vi "XY Dialog - Update FP Settings With Persistent Data.vi"(7 "GraphData.System.Root":refnum<k24>, 8 "error in (no error)":errorcluster, 10 "References":T9, 11 "Persistent Data":T1={"Label"="", "Graph Props"={"Plots"=[], "Legend:Number of Rows"=0, "Scale Properties"={"X.Auto"=FALSE, "X.Min"=0.0, "X.Max"=0.0, "X.IgnoreTS"=FALSE, "X.Precision"=0, "X.Label:"="", "X.LabelVis"=FALSE, "X.DefLabel"=FALSE, "Y.Auto"=FALSE, "Y.Min"=0.0, "Y.Max"=0.0, "Y.Format"=0, "Y.Precision:"=0, "Y.Label:"="", "Y.LabelVis"=FALSE, "Y.DefLabel"=FALSE, "X.Format"=0}, "Legend:Visible"=TRUE, "BgColor"=0, "Last Plot Width"=0, "Resize"=FALSE}, "UDP Data"={"Decimation"=0, "UDP Buffer Size"=0, "History Length"=0.0, "Update Rate"=enum."15 Hz", "Channel Paths"=[], "Channel Names"=[]}} {"Graph Props"."Scale Properties"."X.Format" items=["Decimal", "Scientific", "Engineering", "Binary", "Octal", "Hexadecimal", "Relative Time", "Time and Date", "SI", "Automatic"]; "Graph Props"."Scale Properties"."Y.Precision:" items=["0", "1", "2", "3", "4", "5", "6", "7"]; "Graph Props"."Scale Properties"."Y.Format" items=["Decimal", "Scientific", "Engineering", "Binary", "Octal", "Hexadecimal", "Relative Time", "Time and Date", "SI", "Automatic"]; "Graph Props"."Scale Properties"."X.Precision" items=["0", "1", "2", "3", "4", "5", "6", "7"]}) -> (0 "error out":errorcluster)   [LabVIEW 2020, in "Workspace MultiY Graph.lvlib"]
uses:
  Workspace MultiY Graph.lvlib
  XY Dialog References.ctl
  XY Scale Precision.ctl
  XY Scale Format.ctl
  XY Persistent Data.ctl
  XY Graph Properties.ctl
  XY Plot Properties.ctl
  XY Scale Properties.ctl
  UDP Data.ctl
  Update Rate.ctl
  NationalInstruments.VeriStand.SystemStorage
  NationalInstruments.VeriStand
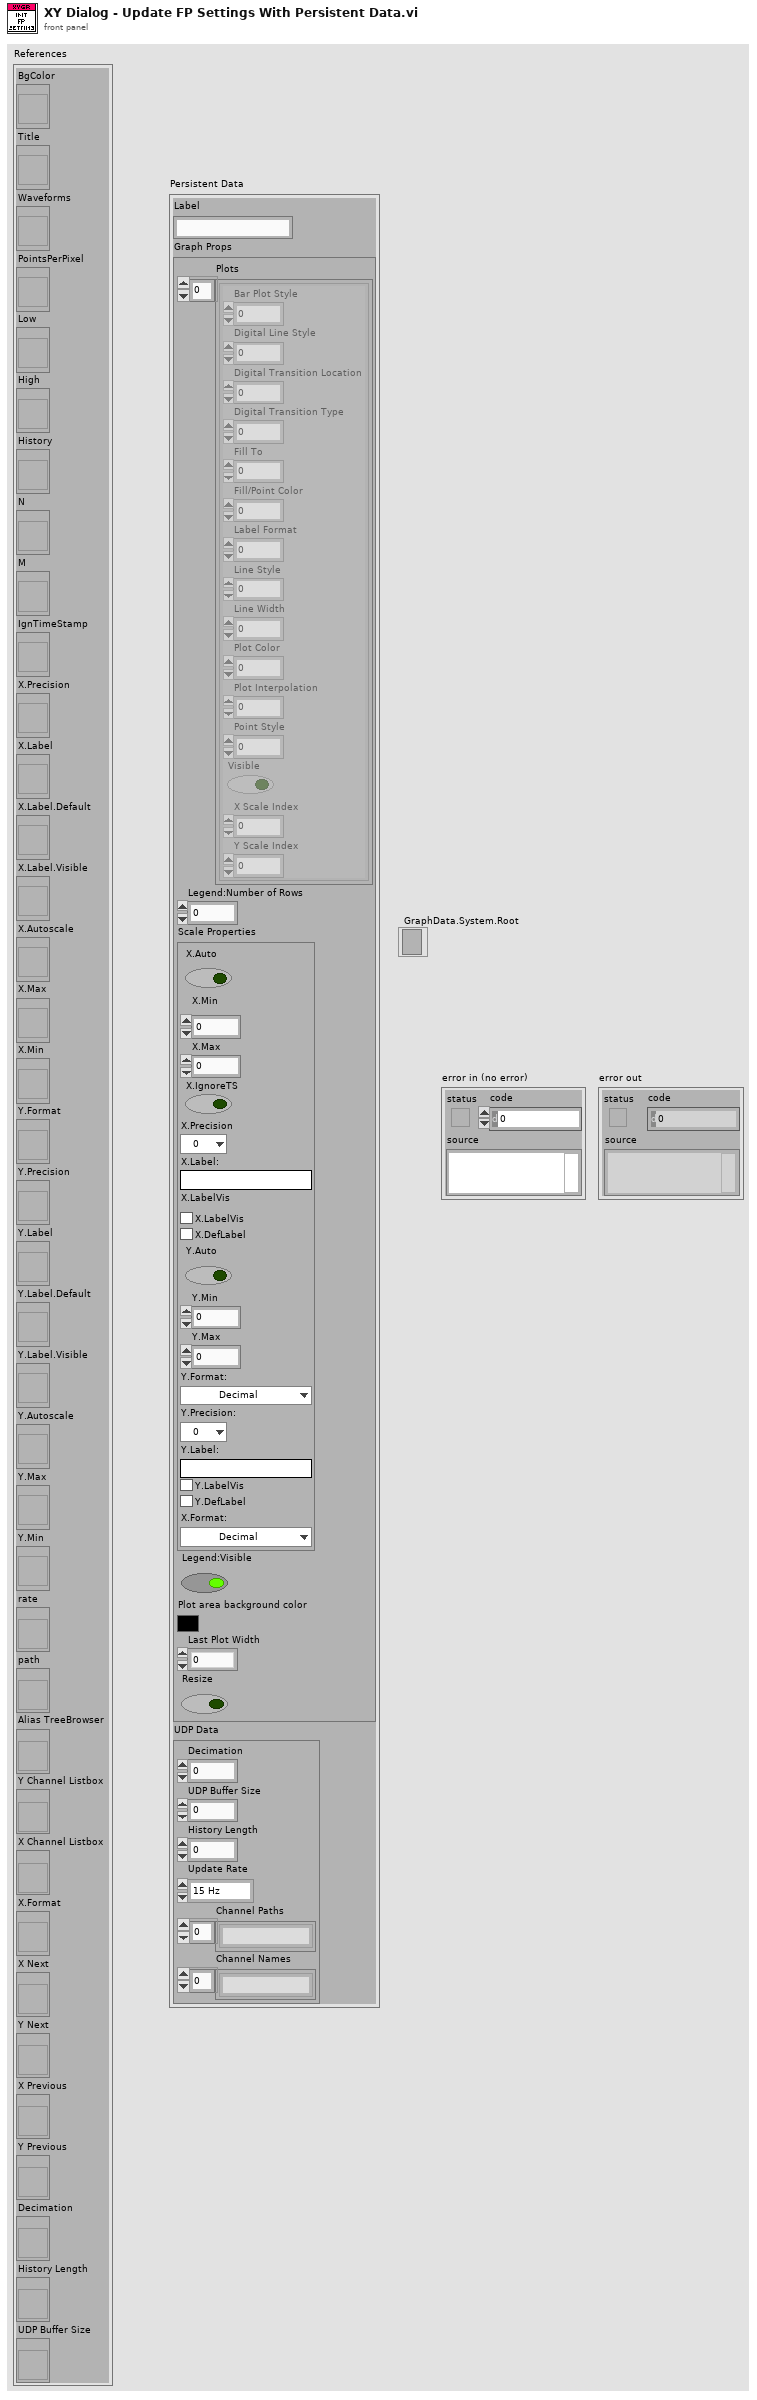
[diagram p1: front panel]
types:
  T1 = typedef "Workspace MultiY Graph.lvlib/XY Persistent Data.ctl" = cluster{"Label":string, "Graph Props":T2, "UDP Data":T7}
  T2 = typedef "Workspace MultiY Graph.lvlib/XY Graph Properties.ctl" = cluster{"Plots":T3[], "Legend:Number of Rows":u32, "Scale Properties":T4, "Legend:Visible":bool, "BgColor":u32, "Last Plot Width":u32, "Resize":bool}
  T3 = typedef "Workspace MultiY Graph.lvlib/XY Plot Properties.ctl" = cluster{"Bar Plot Style":u8, "Digital Line Style":u8, "Digital Transition Location":u8, "Digital Transition Type":u8, "Fill To":i16, "Fill/Point Color":u32, "Label Format":u8, "Line Style":u8, "Line Width":u8, "Plot Color":u32, "Plot Interpolation":u8, "Point Style":u8, "Visible":bool, "X Scale Index":u32, "Y Scale Index":u32}
  T4 = typedef "Workspace MultiY Graph.lvlib/XY Scale Properties.ctl" = cluster{"X.Auto":bool, "X.Min":dbl, "X.Max":dbl, "X.IgnoreTS":bool, "X.Precision":T5, "X.Label:":string, "X.LabelVis":bool, "X.DefLabel":bool, "Y.Auto":bool, "Y.Min":dbl, "Y.Max":dbl, "Y.Format":T6, "Y.Precision:":T5, "Y.Label:":string, "Y.LabelVis":bool, "Y.DefLabel":bool, "X.Format":T6}
  T5 = typedef "Workspace MultiY Graph.lvlib/XY Scale Precision.ctl" = u8
  T6 = typedef "Workspace MultiY Graph.lvlib/XY Scale Format.ctl" = u8
  T7 = typedef "Workspace MultiY Graph.lvlib/UDP Data.ctl" = cluster{"Decimation":i32, "UDP Buffer Size":u32, "History Length":dbl, "Update Rate":T8, "Channel Paths":string[], "Channel Names":string[]}
  T8 = typedef "Workspace MultiY Graph.lvlib/Update Rate.ctl" = enum8{"15 Hz", "10 Hz", "5 Hz", "4 Hz", "3 Hz", "2 Hz", "1 Hz", "0.5 Hz"}
  T9 = typedef "Workspace MultiY Graph.lvlib/XY Dialog References.ctl" = cluster{"BgColor":refnum<vi>, "Title":refnum<vi>, "Waveforms":refnum<vi>, "PointsPerPixel":refnum<vi>, "Low":refnum<vi>, "High":refnum<vi>, "History":refnum<vi>, "N":refnum<vi>, "M":refnum<vi>, "IgnTimeStamp":refnum<vi>, "X.Precision":refnum<vi>, "X.Label":refnum<vi>, "X.Label.Default":refnum<vi>, "X.Label.Visible":refnum<vi>, "X.Autoscale":refnum<vi>, "X.Max":refnum<vi>, "X.Min":refnum<vi>, "Y.Format":refnum<vi>, "Y.Precision":refnum<vi>, "Y.Label":refnum<vi>, "Y.Label.Default":refnum<vi>, "Y.Label.Visible":refnum<vi>, "Y.Autoscale":refnum<vi>, "Y.Max":refnum<vi>, "Y.Min":refnum<vi>, "rate":refnum<vi>, "path":refnum<vi>, "Alias TreeBrowser":refnum<vi>, "Y Channel Listbox":refnum<vi>, "X Channel Listbox":refnum<vi>, "X.Format":refnum<vi>, "X Next":refnum<vi>, "Y Next":refnum<vi>, "X Previous":refnum<vi>, "Y Previous":refnum<vi>, "Decimation":refnum<vi>, "History Length":refnum<vi>, "UDP Buffer Size":refnum<vi>}
  T10 = enum8{"Enabled", "Disabled", "Disabled and Grayed Out"}
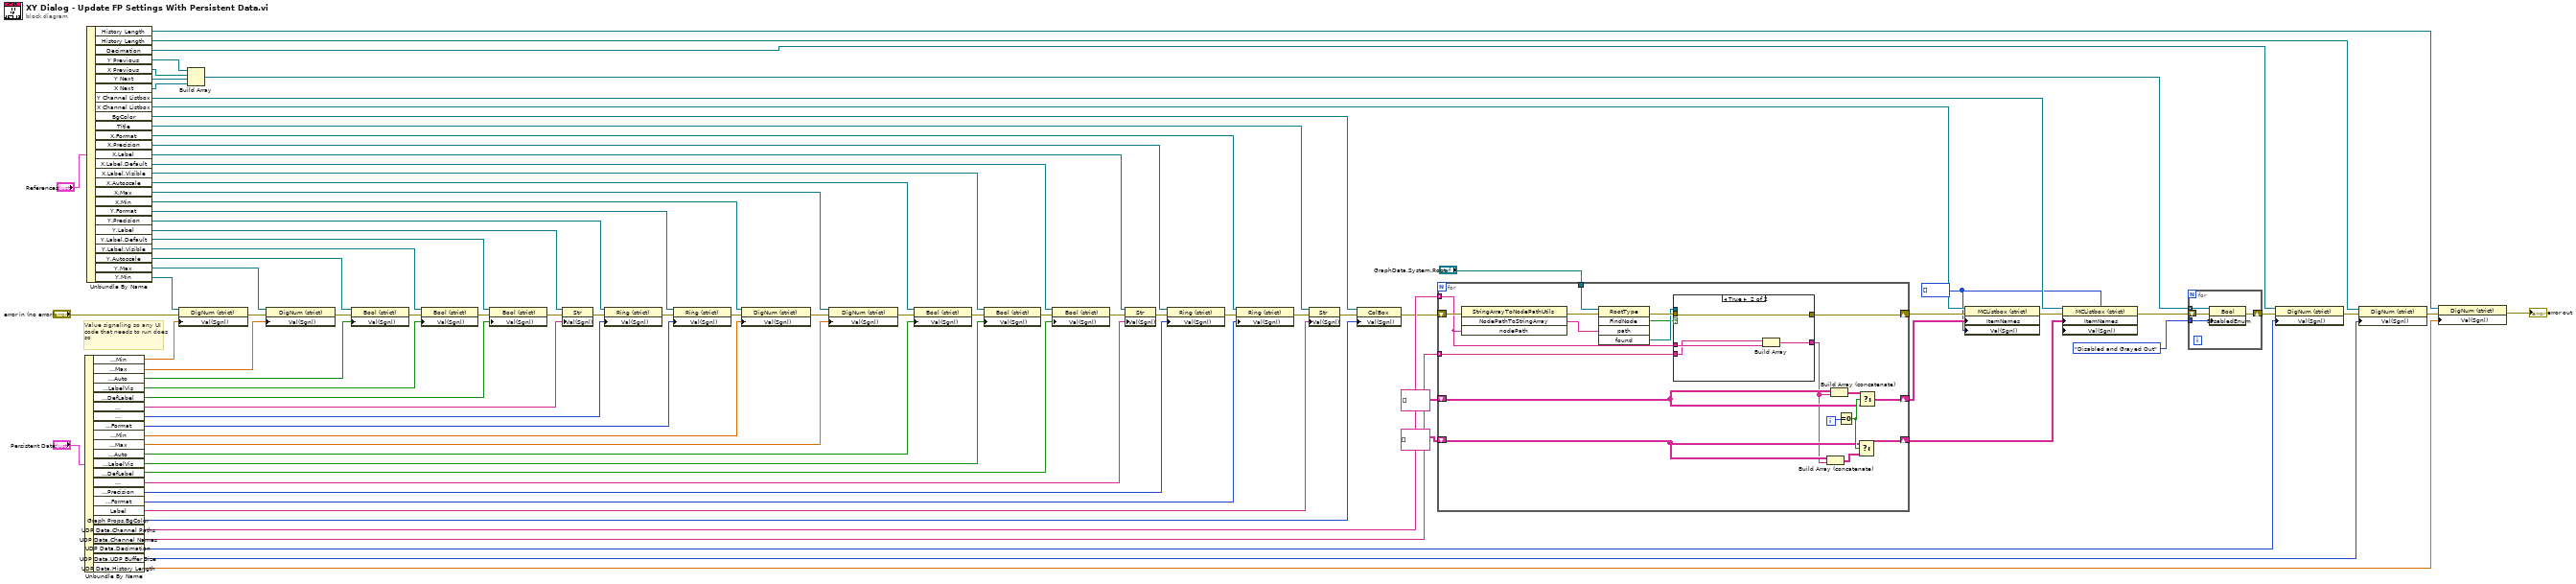
[diagram p0: block diagram]
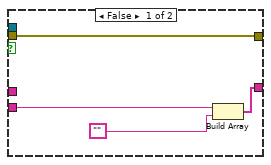
[diagram p2: hidden frame]
diagram:
  w23 = i32[] [] ("Value (Signaling)")
  # "Value signaling so any UI code that needs to run does so"
  n1 = Unbundle By Name("Persistent Data") -> ("Graph Props.Scale Properties.Y.Min"=w80:dbl, "Graph Props.Scale Properties.Y.Max"=w79:dbl, "Graph Props.Scale Properties.Y.Auto"=w76:bool, "Graph Props.Scale Properties.Y.LabelVis"=w73:bool, "Graph Props.Scale Properties.Y.DefLabel"=w70:bool, "Graph Props.Scale Properties.Y.Label:"=w67:string, "Graph Props.Scale Properties.Y.Precision:"=w64:T5, "Graph Props.Scale Properties.Y.Format"=w61:T6, "Graph Props.Scale Properties.X.Min"=w46:dbl, "Graph Props.Scale Properties.X.Max"=w45:dbl, "Graph Props.Scale Properties.X.Auto"=w44:bool, "Graph Props.Scale Properties.X.LabelVis"=w43:bool, "Graph Props.Scale Properties.X.DefLabel"=w42:bool, "Graph Props.Scale Properties.X.Label:"=w41:string, "Graph Props.Scale Properties.X.Precision"=w40:T5, "Graph Props.Scale Properties.X.Format"=w2:T6, "Label"=w38:string, "Graph Props.BgColor"=w35:u32, "UDP Data.Channel Paths"=w31:string[], "UDP Data.Channel Names"=w5:string[], "UDP Data.Decimation"=w8:i32, "UDP Data.UDP Buffer Size"=w7:u32, "UDP Data.History Length"=w6:dbl)
  n2 = Unbundle By Name("References") -> ("History Length"=w10:refnum<vi>, "History Length"=w12:refnum<vi>, "Decimation"=w14:refnum<vi>, "Y Previous"=w20:refnum<vi>, "X Previous"=w19:refnum<vi>, "Y Next"=w18:refnum<vi>, "X Next"=w17:refnum<vi>, "Y Channel Listbox"=w33:refnum<vi>, "X Channel Listbox"=w34:refnum<vi>, "BgColor"=w36:refnum<vi>, "Title"=w39:refnum<vi>, "X.Format"=w1:refnum<vi>, "X.Precision"=w47:refnum<vi>, "X.Label"=w48:refnum<vi>, "X.Label.Default"=w49:refnum<vi>, "X.Label.Visible"=w50:refnum<vi>, "X.Autoscale"=w51:refnum<vi>, "X.Max"=w52:refnum<vi>, "X.Min"=w53:refnum<vi>, "Y.Format"=w62:refnum<vi>, "Y.Precision"=w65:refnum<vi>, "Y.Label"=w68:refnum<vi>, "Y.Label.Default"=w71:refnum<vi>, "Y.Label.Visible"=w74:refnum<vi>, "Y.Autoscale"=w77:refnum<vi>, "Y.Max"=w81:refnum<vi>, "Y.Min"=w83:refnum<vi>)
  n3 = property class="DigNum (strict)"(reference=w83, error in="error in (no error)", "Val(Sgnl)"=w80) -> (error out=w82:errorcluster)  [unwired: 1 out]
  n4 = Build Array(w20, w19, w18, w17) -> (w16:refnum<vi>[])
  n5 = property class="DigNum (strict)"(reference=w81, error in=w82, "Val(Sgnl)"=w79) -> (error out=w78:errorcluster)  [unwired: 1 out]
  n6 = property class="Bool (strict)"(reference=w77, error in=w78, "Val(Sgnl)"=w76) -> (error out=w75:errorcluster)  [unwired: 1 out]
  n7 = property class="Bool (strict)"(reference=w74, error in=w75, "Val(Sgnl)"=w73) -> (error out=w72:errorcluster)  [unwired: 1 out]
  n8 = property class="Bool (strict)"(reference=w71, error in=w72, "Val(Sgnl)"=w70) -> (error out=w69:errorcluster)  [unwired: 1 out]
  n9 = property class="Str"(reference=w68, error in=w69, "Val(Sgnl)"=w67) -> (error out=w66:errorcluster)  [unwired: 1 out]
  n10 = property class="Ring (strict)"(reference=w65, error in=w66, "Val(Sgnl)"=w64) -> (error out=w63:errorcluster)  [unwired: 1 out]
  n11 = property class="Ring (strict)"(reference=w62, error in=w63, "Val(Sgnl)"=w61) -> (error out=w54:errorcluster)  [unwired: 1 out]
  n12 = property class="DigNum (strict)"(reference=w53, error in=w54, "Val(Sgnl)"=w46) -> (error out=w55:errorcluster)  [unwired: 1 out]
  n13 = property class="DigNum (strict)"(reference=w52, error in=w55, "Val(Sgnl)"=w45) -> (error out=w56:errorcluster)  [unwired: 1 out]
  n14 = property class="Bool (strict)"(reference=w51, error in=w56, "Val(Sgnl)"=w44) -> (error out=w57:errorcluster)  [unwired: 1 out]
  n15 = property class="Bool (strict)"(reference=w50, error in=w57, "Val(Sgnl)"=w43) -> (error out=w58:errorcluster)  [unwired: 1 out]
  n16 = property class="Bool (strict)"(reference=w49, error in=w58, "Val(Sgnl)"=w42) -> (error out=w59:errorcluster)  [unwired: 1 out]
  n17 = property class="Str"(reference=w48, error in=w59, "Val(Sgnl)"=w41) -> (error out=w60:errorcluster)  [unwired: 1 out]
  n18 = property class="Ring (strict)"(reference=w47, error in=w60, "Val(Sgnl)"=w40) -> (error out=w4:errorcluster)  [unwired: 1 out]
  n19 = property class="Ring (strict)"(reference=w1, error in=w4, "Val(Sgnl)"=w2) -> (error out=w3:errorcluster)  [unwired: 1 out]
  n20 = property class="Str"(reference=w39, error in=w3, "Val(Sgnl)"=w38) -> (error out=w37:errorcluster)  [unwired: 1 out]
  n21 = property class="ColBox"(reference=w36, error in=w37, "Val(Sgnl)"=w35) -> (error out=w29:errorcluster)  [unwired: 1 out]
  n22 = for {
    tunnel: "GraphData.System.Root" -> [w105]
    shift-right: [w99] -> w28
    shift-left: w29 -> [w104]
    tunnel: w31 -> [w92] mode=indexing
    shift-right: [w95] -> w24
    shift-left: string[][] [] -> [w96]
    shift-right: [w93] -> w25
    shift-left: string[][] [] -> [w94]
    tunnel: w5 -> [w87] mode=indexing
    i -> [w98]
    n23 = invoke class="StringArrayToNodePathUtils" method="NodePathToStringArray"(error in=w104, "nodePath"=w92) -> (error out=w103:errorcluster, "NodePathToStringArray"=w102:string[])  [unwired: 2 in, 2 out]
    n24 = invoke class="RootType" method="FindNode"(reference=w105, error in=w103, "path"=w102) -> (error out=w101:errorcluster, "FindNode"=w88:bool, "found"=w100:refnum<k24>)  [unwired: 2 in, 2 out]
    n25 = case shown="True" w88 {
      tunnel: w101 -> [w107 w110]
      tunnel: w100 -> [_ _]
      tunnel: [w107 w110] -> w99
      tunnel: w92 -> [_ w113]
      tunnel: [w108 w112] -> w90
      tunnel: w87 -> [w106 w111]
      frame False {
        n26 = Build Array(w106, "") -> (w108:string[])
      }
      frame True {
        n27 = Build Array(w111, w113) -> (w112:string[])
      }
    }
    n28 = Build Array (concatenate)(w96, w90) -> (w91:string[][])
    n29 = Build Array (concatenate)(w94, w90) -> (w89:string[][])
    n30 = Equal To 0?(x=w98) -> (x = 0?=w97:bool)
    n31 = Select(t=w96, s=w97, f=w91) -> (s? t:f=w95:string[][])
    n32 = Select(t=w89, s=w97, f=w94) -> (s? t:f=w93:string[][])
  }
  n33 = property class="MCListbox (strict)"(reference=w34, error in=w28, "ItemNames"=w25, "Val(Sgnl)"=w23) -> (error out=w32:errorcluster)  [unwired: 1 out]
  n34 = property class="MCListbox (strict)"(reference=w33, error in=w32, "ItemNames"=w24, "Val(Sgnl)"=w23) -> (error out=w22:errorcluster)  [unwired: 1 out]
  n35 = for {
    tunnel: T10."Disabled and Grayed Out" ("Disabled") -> [w116]
    tunnel: w16 -> [w114] mode=indexing
    shift-right: [w115] -> w15
    shift-left: w22 -> [w117]
    n36 = property class="Bool"(reference=w114, error in=w117, "DisabledEnum"=w116) -> (error out=w115:errorcluster)  [unwired: 1 out]
  }
  n37 = property class="DigNum (strict)"(reference=w14, error in=w15, "Val(Sgnl)"=w8) -> (error out=w13:errorcluster)  [unwired: 1 out]
  n38 = property class="DigNum (strict)"(reference=w12, error in=w13, "Val(Sgnl)"=w7) -> (error out=w11:errorcluster)  [unwired: 1 out]
  n39 = property class="DigNum (strict)"(reference=w10, error in=w11, "Val(Sgnl)"=w6) -> (error out=→"error out":errorcluster)  [unwired: 1 out]
